vi "Yokogawa WT300 Series Measure Normal Preset.vi"() -> ()   [LabVIEW 2019]
doc: "This example shows how to measure the normal numeric preset data."
uses:
  Public/Data/Read Measurement (Normal).vi
  Yokogawa WT300 Series.lvlib
panel:
  in  "Preset (1:Pattern 1)":i32(ring)=1 items=["Pattern 1"=1, "Pattern 2"=2, "Pattern 3"=3, "Pattern 4"=4]
  out "Function":string[](array[string])
  out "Measurement":dbl[](array[numeric])
  in  "Number of Item (10)":i32=10 min=1 max=255
  in  "Timeout (10000 ms)":i32=10000 min=1
  in  "VISA resource name":refnum<visa-resource-name>
  # "(c) 2013 Yokogawa Meters & Instruments Corporation.  All rights reserved."
  # "WT300 SERIES POWER ANALYZER"
  # "ms"
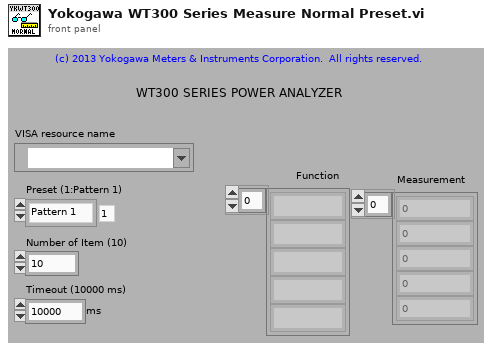
[diagram p1: front panel]
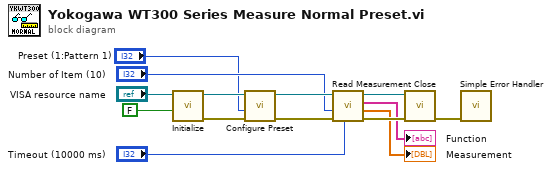
[diagram p0: block diagram]
diagram:
  n1 = call "Initialize.vi"("Reset (True)"=FALSE ("Reset? (True)"), "VISA resource name"="VISA resource name") -> ("error out"=w2:errorcluster, "VISA resource name out"=w3:refnum<visa-resource-name>)  [unwired: 7 in, 1 out]
  n2 = call "Configure Preset.vi"("error in (no error)"=w2, "Preset (1:Pattern 1)"="Preset (1:Pattern 1)", "VISA resource name"=w3) -> ("error out"=w8:errorcluster, "VISA resource name out"=w9:refnum<visa-resource-name>)  [unwired: 7 in]
  n3 = call-poly "Read Measurement.vi"("Timeout (10000 ms)"="Timeout (10000 ms)", "error in (no error)"=w8, "Number of Item (15)"="Number of Item (10)", "VISA resource name"=w9) -> ("error out"=w11:errorcluster, "Measurement"=→"Measurement":dbl[], "Function"=→"Function":string[], "VISA resource name out"=w12:refnum<visa-resource-name>)  [unwired: 4 in]
  n4 = call "Close.vi"("error in (no error)"=w11, "VISA resource name"=w12) -> ("error out"=w14:errorcluster)  [unwired: 9 in]
  n5 = call <vilib>:"Simple Error Handler.vi"("error in (no error)"=w14) -> ()  [unwired: 4 in, 5 out]
